vi "SHI_Cryopump_interface_GUI.vi"(8 "error in (no error)":errorcluster, 9 "URL prefex":string, 10 "Http session":T1, 11 "go":bool=TRUE) -> ()   [LabVIEW 2017]
uses:
  Type_Defs/Cryo_Pump_MCC_Status.ctl
  Type_Defs/Cryo_Pump_MCC_CryoPump.ctl
  Type_Defs/Cryo_Pump_MCC_RoughingInterlock.ctl
  Type_Defs/Cryo_Pump_MCC_Status_Status.ctl
  Type_Defs/Cryo_Pump_MCC_Start_Regen.ctl
  Type_Defs/Cryo_Pump_MCC_First_Stage_Temp_CTL.ctl
  Type_Defs/Cryo_Pump_MCC_Params_Power_Failure_Recovery.ctl
  Type_Defs/Cryo_Pump_MCC_Regen_Params.ctl
  Type_Defs/Cryo_Pump_Compressor_Status.ctl
  Type_Defs/Cryo_Pump_Compressor_Status_Status.ctl
  <vilib>/httpClient/ClientHandle.ctl
  Type_Defs/Cryo_Pump_Plots.ctl
  Type_Defs/Cryo_Pump_MCC_Params.ctl
  msg7171_linux.llb/send single message.vi
  msg7171_linux.llb/send multiple messages.vi
  <vilib>/httpClient/POSTBuffer.vi
  <vilib>/httpClient/LabVIEWHTTPClient.lvlib
panel:
  in  "Cold Head Start":bool
  in  "Compressor On":bool
  in  "Roughing_Ilock_Permission":bool
  in  "TC_Pressure_Guage":bool
  in  "Roughing Valve":bool
  in  "Purge Valve":bool
  in  "Send Regen Start":bool
  out "Compressor":T2
  in  "2nd Stage Temp CTL":u32 max=320 step=1
  out "Regen Time":u32
  out "Regen Step Timer":u32
  in  "Regen Start Delay":u32 max=59994 step=1
  in  "Regen Parameters":T4 {"z" max=1 step=1; "G" max=9999 step=1; "C" min=1 max=3 step=1; "A" max=1 step=1; "6" max=80 step=1; "5" max=200 step=1; "4" min=1 max=100 step=1; "3" min=25 max=200 step=1; "2" max=200 step=1; "1" max=9990 step=1; "0" max=59994 step=1}
  out "Regen Cycles":u32
  out "Power Failure Recovery Status":string
  in  "Power Failure Recovery":T5 items=["Disabled", "Enabled", "Enabled only when Stage 2 < Restart Temp."]
  out "MCC Version":string
  out "Last Rate Of Rise Value":u32
  in  "1st Stage Temp Ctl":T6 {"method" items=["ExtHeat", "1st s ctl", "2nd sctl", "Dual"]; "temp" max=320 step=1}
  out "Failed Repurge Cycles":u32
  out "Failed Rate Of Rise Cycles":u32
  out "Elapsed Time":u32
  in  "Start Regen Parameter":T7=enum."Start full regeneration cycle"
  out "MCC Status":T8
  out "Get Params json":string
  out "Get Status json":string
  in  "exit":bool
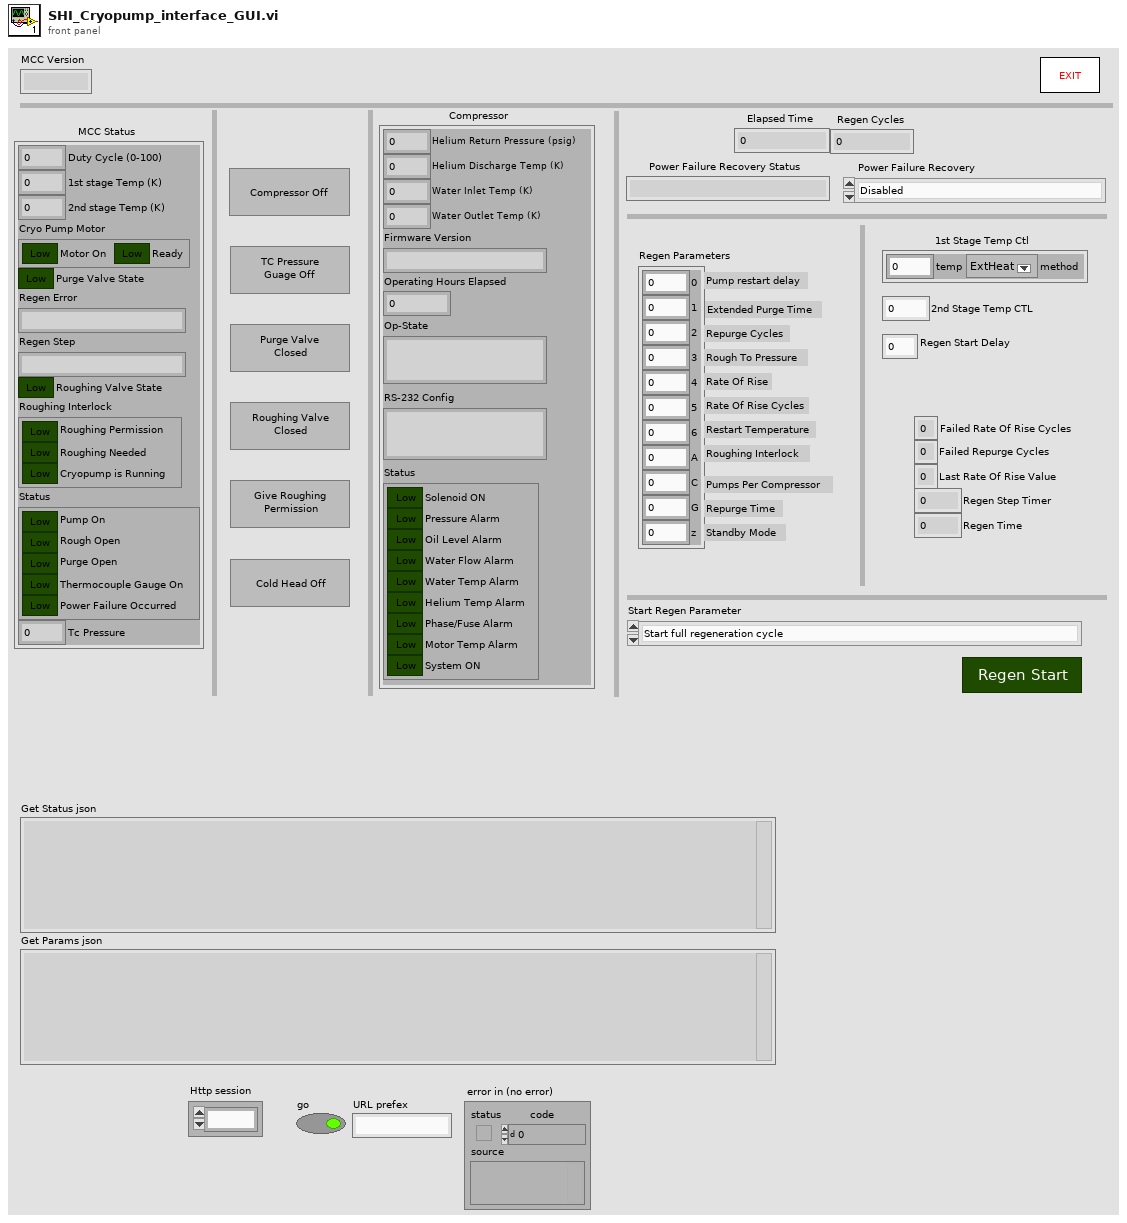
[diagram p1: front panel]
types:
  T1 = typedef "LabVIEWHTTPClient.lvlib/ClientHandle.ctl" = refnum<k1>
  T2 = typedef "Cryo_Pump_Compressor_Status.ctl" = cluster{"Helium Return Pressure (psig)":u32, "Helium Discharge Temp (K)":u32, "Water Inlet Temp (K)":u32, "Water Outlet Temp (K)":u32, "Firmware Version":string, "Operating Hours Elapsed":dbl, "Op-State":string, "RS-232 Config":string, "Status":T3}
  T3 = typedef "Cryo_Pump_Compressor_Status_Status.ctl" = cluster{"Solenoid ON":bool, "Pressure Alarm":bool, "Oil Level Alarm":bool, "Water Flow Alarm":bool, "Water Temp Alarm":bool, "Helium Temp Alarm":bool, "Phase/Fuse Alarm":bool, "Motor Temp Alarm":bool, "System ON":bool}
  T4 = typedef "Cryo_Pump_MCC_Regen_Params.ctl" = cluster{"0":u32, "1":u32, "2":u32, "3":u32, "4":u32, "5":u32, "6":u32, "A":u32, "C":u32, "G":u32, "z":u32}
  T5 = typedef "Cryo_Pump_MCC_Params_Power_Failure_Recovery.ctl" = u16
  T6 = typedef "Cryo_Pump_MCC_First_Stage_Temp_CTL.ctl" = cluster{"temp":u32, "method":u32}
  T7 = typedef "Cryo_Pump_MCC_Start_Regen.ctl" = enum16{"Abort current regeneration cycle", "Start full regeneration cycle", "Start fast regeneration cycle", "Activate stand-by pump module for normal pumping operation", "Warm up cryopump and stop"}
  T8 = typedef "Cryo_Pump_MCC_Status.ctl" = cluster{"Duty Cycle (0-100)":dbl, "1st stage Temp (K)":dbl, "2nd stage Temp (K)":dbl, "Cryo Pump Motor":T9, "Purge Valve State":bool, "Regen Error":string, "Regen Step":string, "Roughing Valve State":bool, "Roughing Interlock":T10, "Status":T11, "Tc Pressure":dbl}
  T9 = typedef "Cryo_Pump_MCC_CryoPump.ctl" = cluster{"Motor On":bool, "Ready":bool}
  T10 = typedef "Cryo_Pump_MCC_RoughingInterlock.ctl" = cluster{"Roughing Permission":bool, "Roughing Needed":bool, "Cryopump is Running":bool}
  T11 = typedef "Cryo_Pump_MCC_Status_Status.ctl" = cluster{"Pump On":bool, "Rough Open":bool, "Purge Open":bool, "Thermocouple Gauge On":bool, "Power Failure Occurred":bool}
  T12 = typedef "Cryo_Pump_Plots.ctl" = cluster{"Duty Cycle (0-100)":dbl, "1st stage Temp (K)":dbl, "2nd stage Temp (K)":dbl, "Helium Return Pressure (psig)":u32, "Helium Discharge Temp (C)":u32, "Water Inlet Temp (C)":u32, "Water Outlet Temp (C)":u32}
  T13 = cluster{"go":bool, "Http session":T1, "URL prefex":string, "Next get param":u32}
  T14 = typedef "Cryo_Pump_MCC_Params.ctl" = cluster{"MCC Version":string, "First Stage Temp CTL":T6, "Second Stage Temp CTL":u32, "Tc Pressure State":bool, "Elapsed Time":u32, "Power Failure Recovery":T5, "Power Failure Recovery Status":string, "Regen Time":u32, "Regen Parameters":T4, "Regen Start Delay":u32, "Regen Step Timer":u32, "Failed Rate Of Rise Cycles":u32, "Failed Repurge Cycles":u32, "Last Rate Of Rise Value":u32, "Regen Cycles":u32}
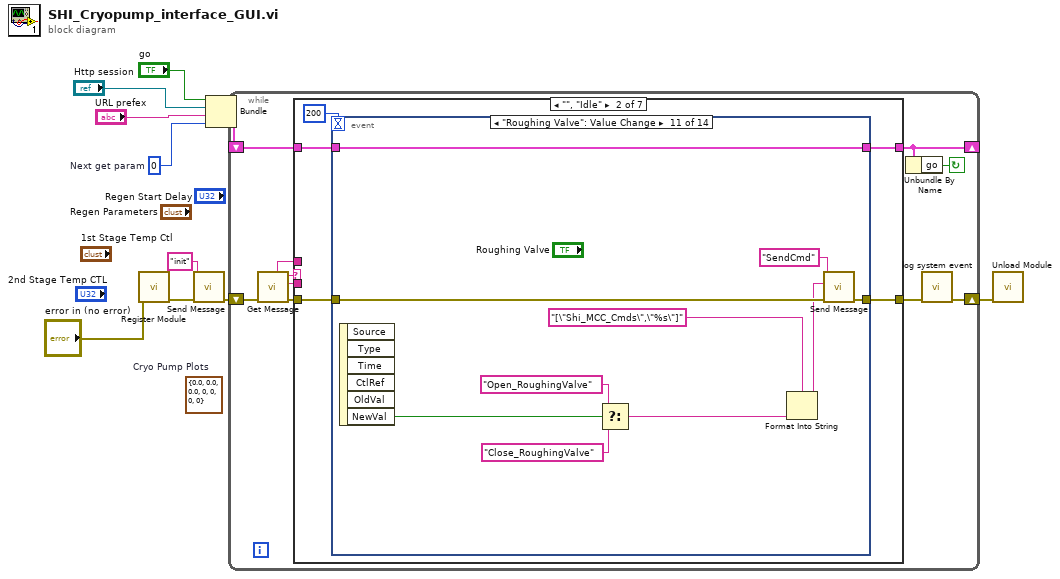
[diagram p0: block diagram]
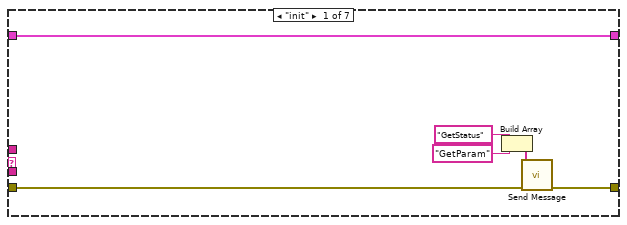
[diagram p2: hidden frame]
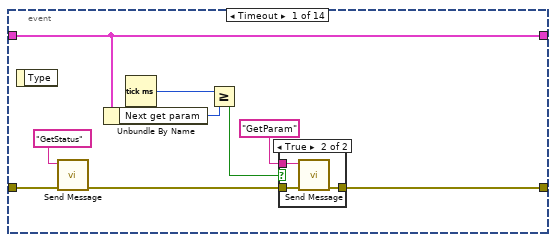
[diagram p3: hidden frame]
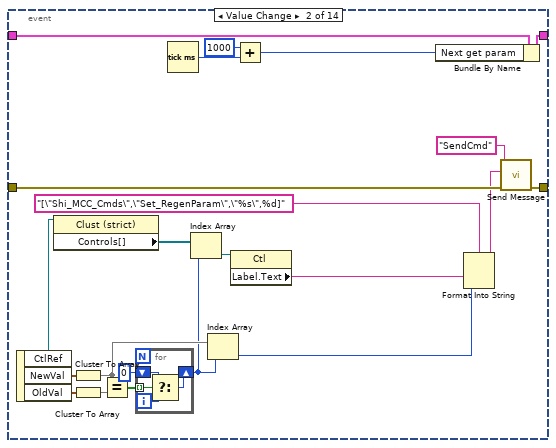
[diagram p5: hidden frame]
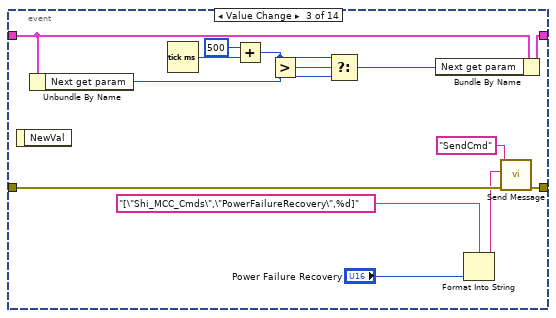
[diagram p6: hidden frame]
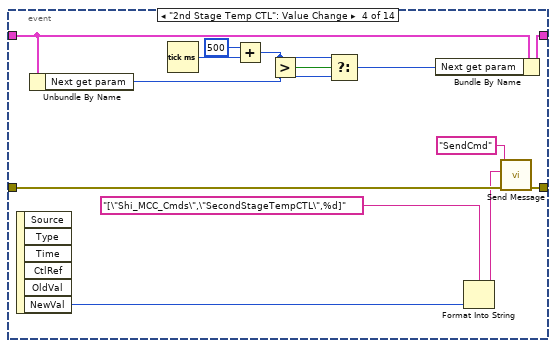
[diagram p7: hidden frame]
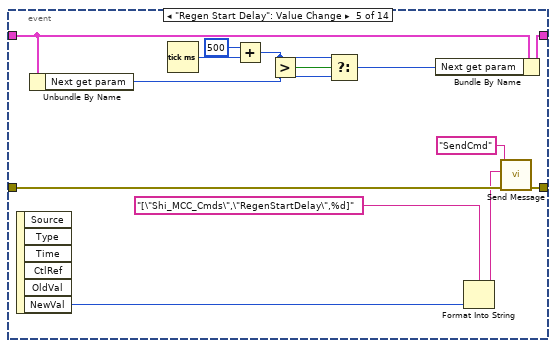
[diagram p8: hidden frame]
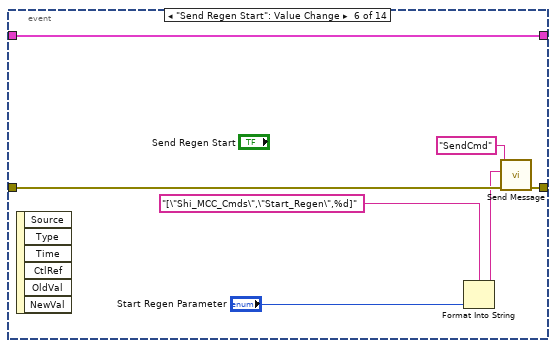
[diagram p9: hidden frame]
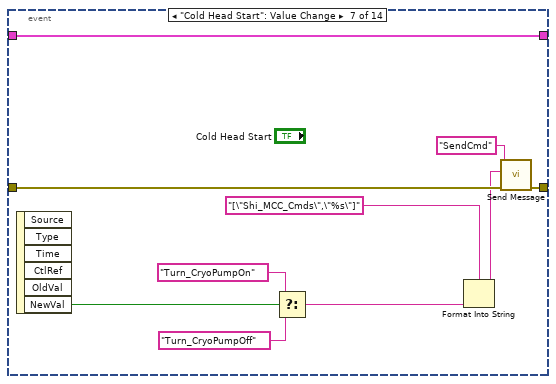
[diagram p10: hidden frame]
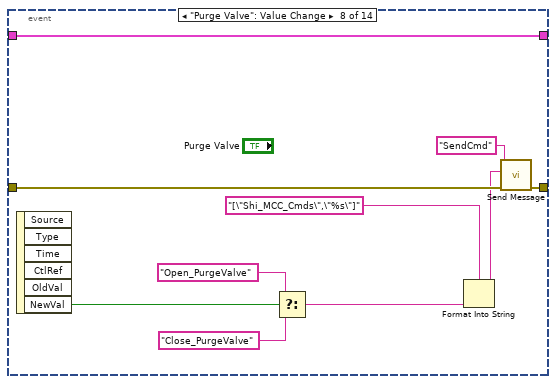
[diagram p11: hidden frame]
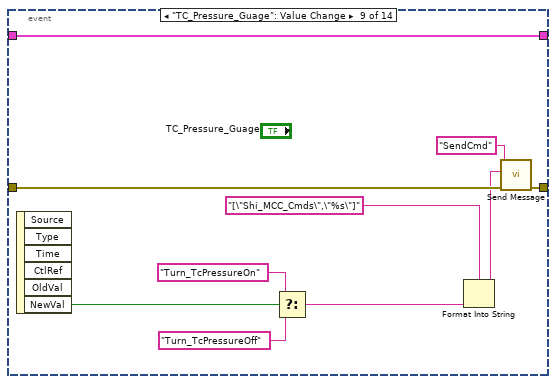
[diagram p12: hidden frame]
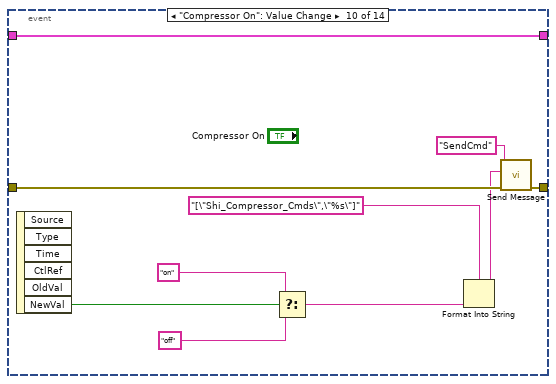
[diagram p13: hidden frame]
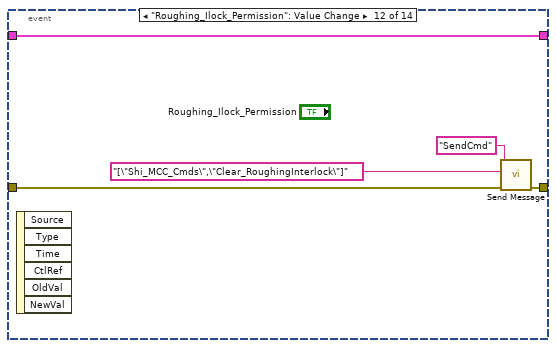
[diagram p14: hidden frame]
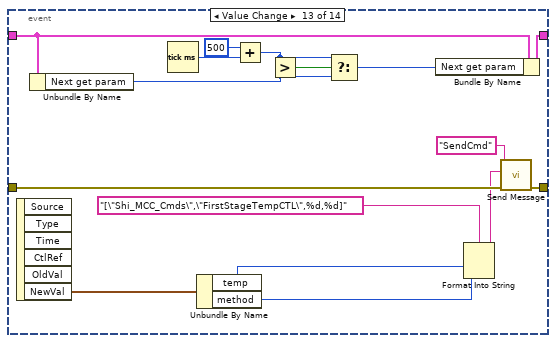
[diagram p15: hidden frame]
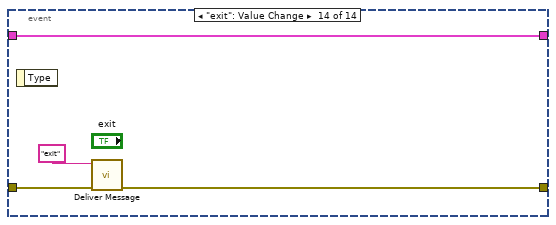
[diagram p16: hidden frame]
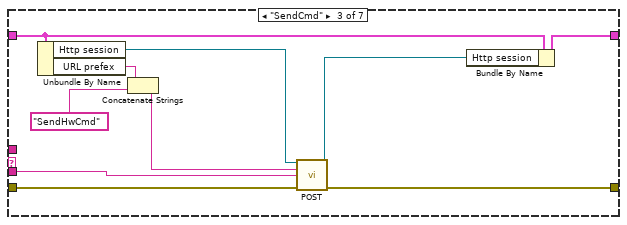
[diagram p17: hidden frame]
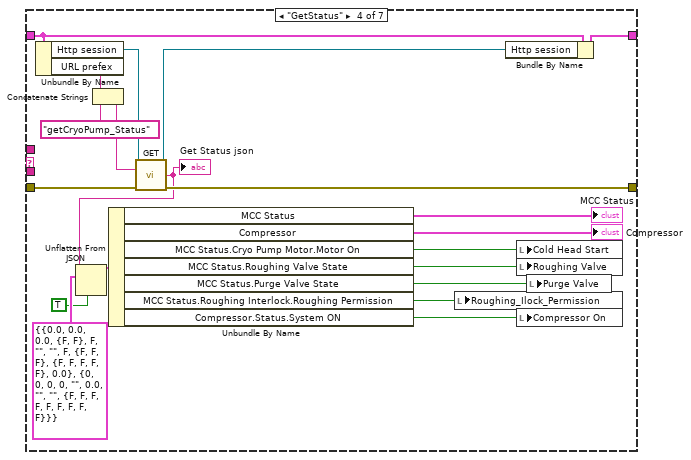
[diagram p18: hidden frame]
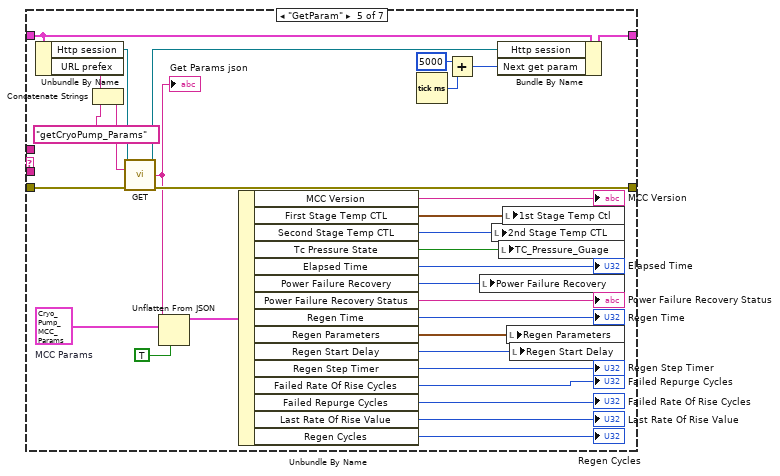
[diagram p19: hidden frame]
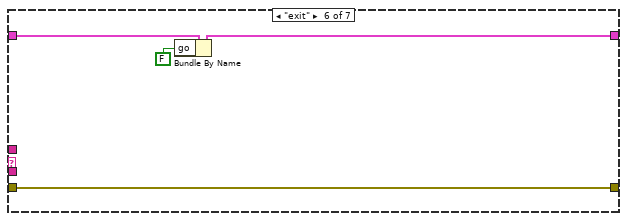
[diagram p20: hidden frame]
diagram:
  (unwired) T12 {"Duty Cycle (0-100)"=0.0, "1st stage Temp (K)"=0.0, "2nd stage Temp (K)"=0.0, "Helium Return Pressure (psig)"=0, "Helium Discharge Temp (C)"=0, "Water Inlet Temp (C)"=0, "Water Outlet Temp (C)"=0}  # Cryo Pump Plots
  w2 = u32 0  # Next get param
  n1 = call "Register Module.vi"("error in (no error)"="error in (no error)") -> ("error out"=w4:errorcluster)  [unwired: 9 in, 1 out]
  n2 = call-poly "Send Message.vi"("error in (no error)"=w4, "event"="init") -> ("error out"=w3:errorcluster)  [unwired: 9 in]
  n3 = Bundle("go"="go", "Http session"="Http session", "URL prefex"="URL prefex", "Next get param"=w2) -> (w10:T13)  [unwired: 1 in]
  n4 = while {
    shift-left: w10 -> [w17]
    shift-right: [w14] -> _
    shift-right: [w12] -> w9
    shift-left: w3 -> [w20]
    stop <- w13 continue-if-true
    n5 = call "Get Message.vi"("error in (no error)"=w20) -> ("error out"=w18:errorcluster, "event buffer"=w19:string, "event"=w16:string, "source"=w15:string)  [unwired: 7 in]
    n6 = case shown="\"\", \"Idle\"" w16 {
      selector: w16 -> [_ _ _ _ _ _ w262]
      tunnel: [w22 w28 w199 w217 w248 w259 w264] -> w14
      tunnel: w17 -> [w22 w27 w198 w216 w247 w257 w264]
      tunnel: w19 -> [_ _ w195 _ _ _ _]
      tunnel: w18 -> [w21 w29 w197 w219 w250 w256 w263]
      tunnel: w15 -> [_ _ _ _ _ _ w261]
      tunnel: [w26 w31 w196 w218 w249 w256 w260] -> w11
      frame "init" {
        n7 = Build Array("GetStatus" ("event"), "GetParam" ("event")) -> (w24:string[])
        n8 = call-poly "Send Message.vi"("error in (no error)"=w21, "event"=w24) -> ("error out"=w26:errorcluster)  [unwired: 9 in]
      }
      frame "", "Idle" {
        n9 = event shown="[10] \"Roughing Valve\": Value Change" {
          selector: _ -> [_ _ _ _ _ _ _ _ _ _ _ _ _ _]
          dyn-events: _ -> [_ _ _ _ _ _ _ _ _ _ _ _ _ _]
          timeout: 200 ("milliseconds to wait") -> [_ _ _ _ _ _ _ _ _ _ _ _ _ _]
          tunnel: w29 -> [w40 w62 w84 w98 w112 w119 w129 w139 w149 w159 w169 w174 w190 w194]
          tunnel: [w36 w61 w83 w97 w111 w118 w128 w138 w148 w158 w168 w173 w189 w193] -> w31
          tunnel: [w32 w48 w78 w92 w106 w113 w120 w130 w140 w150 w160 w170 w184 w191] -> w28
          tunnel: w27 -> [w32 w49 w79 w93 w107 w113 w120 w130 w140 w150 w160 w170 w185 w191]
          event Timeout {
            n10 = event-data() -> ()  [unwired: 1 in, 1 out]
            n11 = call-poly "Send Message.vi"("error in (no error)"=w40, "event"="GetStatus") -> ("error out"=w38:errorcluster)  [unwired: 9 in]
            n12 = Unbundle By Name(w32) -> ("Next get param"=w33:u32)
            n13 = Tick Count (ms)() -> (millisecond timer value=w35:u32)
            n14 = Greater Or Equal?(x=w35, y=w33) -> (x >= y?=w34:bool)
            n15 = case shown="True" w34 {
              tunnel: w38 -> [w41 w44]
              tunnel: [w41 w43] -> w36
              tunnel: "GetParam" ("event") -> [_ w42]
              frame False {
              }
              frame True {
                n16 = call-poly "Send Message.vi"("error in (no error)"=w44, "event"=w42) -> ("error out"=w43:errorcluster)  [unwired: 9 in]
              }
            }
          }
          event Value Change {
            n17 = event-data() -> ("CtlRef"=w53:refnum<vi>, "NewVal"=w63:T4, "OldVal"=w66:T4)  [unwired: 1 in]
            n18 = property class="Clust (strict)"(reference=w53) -> ("Controls[]"=w58:refnum<vi>[])  [unwired: 1 in, 2 out]
            n19 = Cluster To Array(cluster=w63) -> (array=w59:u32[])
            n20 = Cluster To Array(cluster=w66) -> (array=w60:u32[])
            n21 = Equal?(x=w59, y=w60) -> (x = y?=w65:bool[])
            n22 = for {
              tunnel: w65 -> [w70] mode=indexing
              shift-right: [w69] -> w57
              shift-left: 0 -> [w68]
              i -> [w67]
              n23 = Select(t=w68, s=w70, f=w67) -> (s? t:f=w69:i32)
            }
            n24 = Tick Count (ms)() -> (millisecond timer value=w47:u32)
            n25 = Index Array(array=w58, index=w57) -> (element=w56:refnum<vi>)
            n26 = Index Array(array=w59, index=w57) -> (element=w51:u32)
            n27 = property class="Ctl"(reference=w56) -> ("Label.Text"=w50:string)  [unwired: 1 in, 2 out]
            n28 = Add(x=u32 1000, y=w47) -> (x+y=w45:u32)
            n29 = Bundle By Name(cluster=w49, "Next get param"=w45) -> (w48:T13)
            n30 = Format Into String(format string="[\"Shi_MCC_Cmds\",\"Set_RegenParam\",\"%s\",%d]" ("string"), w50, w51) -> (resulting string=w52:string)  [unwired: 2 in, 1 out]
            n31 = call-poly "Send Message.vi"("error in (no error)"=w62, "event buffer"=w52, "event"="SendCmd") -> ("error out"=w61:errorcluster)  [unwired: 8 in]
          }
          event Value Change {
            n32 = event-data() -> ()  [unwired: 1 in, 1 out]
            n33 = Unbundle By Name(w79) -> ("Next get param"=w73:u32)
            n34 = Tick Count (ms)() -> (millisecond timer value=w77:u32)
            n35 = Add(x=u32 500, y=w77) -> (x+y=w72:u32)
            n36 = Greater?(x=w72, y=w73) -> (0:w75:bool)
            n37 = Select(t=w72, s=w75, f=w73) -> (s? t:f=w74:u32)
            n38 = Bundle By Name(cluster=w79, "Next get param"=w74) -> (w78:T13)
            n39 = Format Into String(format string="[\"Shi_MCC_Cmds\",\"PowerFailureRecovery\",%d]" ("string"), "Power Failure Recovery") -> (resulting string=w80:string)  [unwired: 2 in, 1 out]
            n40 = call-poly "Send Message.vi"("error in (no error)"=w84, "event buffer"=w80, "event"="SendCmd") -> ("error out"=w83:errorcluster)  [unwired: 8 in]
          }
          event "2nd Stage Temp CTL": Value Change {
            n41 = event-data() -> ("NewVal"=w85:u32)  [unwired: 1 in, 5 out]
            n42 = Unbundle By Name(w93) -> ("Next get param"=w87:u32)
            n43 = Tick Count (ms)() -> (millisecond timer value=w91:u32)
            n44 = Add(x=u32 500, y=w91) -> (x+y=w86:u32)
            n45 = Greater?(x=w86, y=w87) -> (0:w89:bool)
            n46 = Select(t=w86, s=w89, f=w87) -> (s? t:f=w88:u32)
            n47 = Bundle By Name(cluster=w93, "Next get param"=w88) -> (w92:T13)
            n48 = Format Into String(format string="[\"Shi_MCC_Cmds\",\"SecondStageTempCTL\",%d]" ("string"), w85) -> (resulting string=w94:string)  [unwired: 2 in, 1 out]
            n49 = call-poly "Send Message.vi"("error in (no error)"=w98, "event buffer"=w94, "event"="SendCmd") -> ("error out"=w97:errorcluster)  [unwired: 8 in]
          }
          event "Regen Start Delay": Value Change {
            n50 = event-data() -> ("NewVal"=w99:u32)  [unwired: 1 in, 5 out]
            n51 = Unbundle By Name(w107) -> ("Next get param"=w101:u32)
            n52 = Tick Count (ms)() -> (millisecond timer value=w105:u32)
            n53 = Add(x=u32 500, y=w105) -> (x+y=w100:u32)
            n54 = Greater?(x=w100, y=w101) -> (0:w103:bool)
            n55 = Select(t=w100, s=w103, f=w101) -> (s? t:f=w102:u32)
            n56 = Bundle By Name(cluster=w107, "Next get param"=w102) -> (w106:T13)
            n57 = Format Into String(format string="[\"Shi_MCC_Cmds\",\"RegenStartDelay\",%d]" ("string"), w99) -> (resulting string=w108:string)  [unwired: 2 in, 1 out]
            n58 = call-poly "Send Message.vi"("error in (no error)"=w112, "event buffer"=w108, "event"="SendCmd") -> ("error out"=w111:errorcluster)  [unwired: 8 in]
          }
          event "Send Regen Start": Value Change {
            n59 = event-data() -> ()  [unwired: 1 in, 6 out]
            n60 = Format Into String(format string="[\"Shi_MCC_Cmds\",\"Start_Regen\",%d]" ("string"), "Start Regen Parameter") -> (resulting string=w115:string)  [unwired: 2 in, 1 out]
            n61 = call-poly "Send Message.vi"("error in (no error)"=w119, "event buffer"=w115, "event"="SendCmd") -> ("error out"=w118:errorcluster)  [unwired: 8 in]
          }
          event "Cold Head Start": Value Change {
            n62 = event-data() -> ("NewVal"=w124:bool)  [unwired: 1 in, 5 out]
            n63 = Select(t="Turn_CryoPumpOn", s=w124, f="Turn_CryoPumpOff") -> (s? t:f=w123:string)
            n64 = Format Into String(format string="[\"Shi_MCC_Cmds\",\"%s\"]" ("string"), w123) -> (resulting string=w125:string)  [unwired: 2 in, 1 out]
            n65 = call-poly "Send Message.vi"("error in (no error)"=w129, "event buffer"=w125, "event"="SendCmd") -> ("error out"=w128:errorcluster)  [unwired: 8 in]
          }
          event "Purge Valve": Value Change {
            n66 = event-data() -> ("NewVal"=w134:bool)  [unwired: 1 in, 5 out]
            n67 = Select(t="Open_PurgeValve", s=w134, f="Close_PurgeValve") -> (s? t:f=w133:string)
            n68 = Format Into String(format string="[\"Shi_MCC_Cmds\",\"%s\"]" ("string"), w133) -> (resulting string=w135:string)  [unwired: 2 in, 1 out]
            n69 = call-poly "Send Message.vi"("error in (no error)"=w139, "event buffer"=w135, "event"="SendCmd") -> ("error out"=w138:errorcluster)  [unwired: 8 in]
          }
          event "TC_Pressure_Guage": Value Change {
            n70 = event-data() -> ("NewVal"=w144:bool)  [unwired: 1 in, 5 out]
            n71 = Select(t="Turn_TcPressureOn", s=w144, f="Turn_TcPressureOff") -> (s? t:f=w143:string)
            n72 = Format Into String(format string="[\"Shi_MCC_Cmds\",\"%s\"]" ("string"), w143) -> (resulting string=w145:string)  [unwired: 2 in, 1 out]
            n73 = call-poly "Send Message.vi"("error in (no error)"=w149, "event buffer"=w145, "event"="SendCmd") -> ("error out"=w148:errorcluster)  [unwired: 8 in]
          }
          event "Compressor On": Value Change {
            n74 = event-data() -> ("NewVal"=w154:bool)  [unwired: 1 in, 5 out]
            n75 = Select(t="on", s=w154, f="off") -> (s? t:f=w153:string)
            n76 = Format Into String(format string="[\"Shi_Compressor_Cmds\",\"%s\"]" ("string"), w153) -> (resulting string=w155:string)  [unwired: 2 in, 1 out]
            n77 = call-poly "Send Message.vi"("error in (no error)"=w159, "event buffer"=w155, "event"="SendCmd") -> ("error out"=w158:errorcluster)  [unwired: 8 in]
          }
          event "Roughing Valve": Value Change {
            n78 = event-data() -> ("NewVal"=w164:bool)  [unwired: 1 in, 5 out]
            n79 = Select(t="Open_RoughingValve", s=w164, f="Close_RoughingValve") -> (s? t:f=w163:string)
            n80 = Format Into String(format string="[\"Shi_MCC_Cmds\",\"%s\"]" ("string"), w163) -> (resulting string=w165:string)  [unwired: 2 in, 1 out]
            n81 = call-poly "Send Message.vi"("error in (no error)"=w169, "event buffer"=w165, "event"="SendCmd") -> ("error out"=w168:errorcluster)  [unwired: 8 in]
          }
          event "Roughing_Ilock_Permission": Value Change {
            n82 = event-data() -> ()  [unwired: 1 in, 6 out]
            n83 = call-poly "Send Message.vi"("error in (no error)"=w174, "event buffer"="[\"Shi_MCC_Cmds\",\"Clear_RoughingInterlock\"]" ("string"), "event"="SendCmd") -> ("error out"=w173:errorcluster)  [unwired: 8 in]
          }
          event Value Change {
            n84 = event-data() -> ("NewVal"=w175:T6)  [unwired: 1 in, 5 out]
            n85 = Unbundle By Name(w185) -> ("Next get param"=w179:u32)
            n86 = Tick Count (ms)() -> (millisecond timer value=w183:u32)
            n87 = Unbundle By Name(w175) -> ("temp"=w177:u32, "method"=w176:u32)
            n88 = Add(x=u32 500, y=w183) -> (x+y=w178:u32)
            n89 = Greater?(x=w178, y=w179) -> (0:w181:bool)
            n90 = Select(t=w178, s=w181, f=w179) -> (s? t:f=w180:u32)
            n91 = Bundle By Name(cluster=w185, "Next get param"=w180) -> (w184:T13)
            n92 = Format Into String(format string="[\"Shi_MCC_Cmds\",\"FirstStageTempCTL\",%d,%d]" ("string"), w177, w176) -> (resulting string=w186:string)  [unwired: 2 in, 1 out]
            n93 = call-poly "Send Message.vi"("error in (no error)"=w190, "event buffer"=w186, "event"="SendCmd") -> ("error out"=w189:errorcluster)  [unwired: 8 in]
          }
          event "exit": Value Change {
            n94 = event-data() -> ()  [unwired: 1 in, 1 out]
            n95 = call "Deliver Message.vi"("error in (no error)"=w194, "event"="exit") -> ("error out"=w193:errorcluster)  [unwired: 9 in]
          }
        }
      }
      frame "SendCmd" {
        n96 = Unbundle By Name(w198) -> ("Http session"=w203:T1, "URL prefex"=w201:string)
        n97 = Concatenate Strings(w201, "SendHwCmd" ("url")) -> (w202:string)
        n98 = call-poly <vilib>:"POST.vi"("client handle"=w203, "url"=w202, "buffer"=w195, "error in (no error)"=w197) -> ("client handle out"=w204:T1, "error out"=w196:errorcluster)  [unwired: 8 in, 2 out]
        n99 = Bundle By Name(cluster=w198, "Http session"=w204) -> (w199:T13)
      }
      frame "GetStatus" {
        n100 = Unbundle By Name(w216) -> ("Http session"=w223:T1, "URL prefex"=w221:string)
        n101 = Concatenate Strings(w221, "getCryoPump_Status" ("url")) -> (w222:string)
        n102 = call <vilib>:"GET.vi"("client handle"=w223, "url"=w222, "error in (no error)"=w219) -> ("client handle out"=w224:T1, "body"=w206:string, "error out"=w218:errorcluster)  [unwired: 9 in, 1 out]
        "Get Status json" <- w206
        n103 = Unflatten From JSON(JSON string=w206, type and defaults=cluster{"MCC Status":T8, "Compressor":T2} {"MCC Status"={"Duty Cycle (0-100)"=0.0, "1st stage Temp (K)"=0.0, "2nd stage Temp (K)"=0.0, "Cryo Pump Motor"={"Motor On"=FALSE, "Ready"=FALSE}, "Purge Valve State"=FALSE, "Regen Error"="", "Regen Step"="", "Roughing Valve State"=FALSE, "Roughing Interlock"={"Roughing Permission"=FALSE, "Roughing Needed"=FALSE, "Cryopump is Running"=FALSE}, "Status"={"Pump On"=FALSE, "Rough Open"=FALSE, "Purge Open"=FALSE, "Thermocouple Gauge On"=FALSE, "Power Failure Occurred"=FALSE}, "Tc Pressure"=0.0}, "Compressor"={"Helium Return Pressure (psig)"=0, "Helium Discharge Temp (K)"=0, "Water Inlet Temp (K)"=0, "Water Outlet Temp (K)"=0, "Firmware Version"="", "Operating Hours Elapsed"=0.0, "Op-State"="", "RS-232 Config"="", "Status"={"Solenoid ON"=FALSE, "Pressure Alarm"=FALSE, "Oil Level Alarm"=FALSE, "Water Flow Alarm"=FALSE, "Water Temp Alarm"=FALSE, "Helium Temp Alarm"=FALSE, "Phase/Fuse Alarm"=FALSE, "Motor Temp Alarm"=FALSE, "System ON"=FALSE}}}, default null elements? (F)=TRUE) -> (value=w215:cluster{"MCC Status":T8, "Compressor":T2})  [unwired: 4 in, 1 out]
        n104 = Unbundle By Name(w215) -> ("MCC Status"=→"MCC Status":T8, "Compressor"=→"Compressor":T2, "MCC Status.Cryo Pump Motor.Motor On"=w213:bool, "MCC Status.Roughing Valve State"=w212:bool, "MCC Status.Purge Valve State"=w211:bool, "MCC Status.Roughing Interlock.Roughing Permission"=w210:bool, "Compressor.Status.System ON"=w209:bool)
        n105 = local write "Roughing_Ilock_Permission"(w210) -> ()
        n106 = Bundle By Name(cluster=w216, "Http session"=w224) -> (w217:T13)
        n107 = local write "Cold Head Start"(w213) -> ()
        n108 = local write "Roughing Valve"(w212) -> ()
        n109 = local write "Compressor On"(w209) -> ()
        n110 = local write "Purge Valve"(w211) -> ()
      }
      frame "GetParam" {
        w241 = T14 {"MCC Version"="", "First Stage Temp CTL"={"temp"=0, "method"=0}, "Second Stage Temp CTL"=0, "Tc Pressure State"=FALSE, "Elapsed Time"=0, "Power Failure Recovery"=0, "Power Failure Recovery Status"="", "Regen Time"=0, "Regen Parameters"={"0"=0, "1"=0, "2"=0, "3"=0, "4"=0, "5"=0, "6"=0, "A"=0, "C"=0, "G"=0, "z"=0}, "Regen Start Delay"=0, "Regen Step Timer"=0, "Failed Rate Of Rise Cycles"=0, "Failed Repurge Cycles"=0, "Last Rate Of Rise Value"=0, "Regen Cycles"=0}  # MCC Params
        n111 = Unbundle By Name(w247) -> ("Http session"=w254:T1, "URL prefex"=w252:string)
        n112 = Concatenate Strings(w252, "getCryoPump_Params" ("url")) -> (w253:string)
        n113 = call <vilib>:"GET.vi"("client handle"=w254, "url"=w253, "error in (no error)"=w250) -> ("client handle out"=w255:T1, "body"=w242:string, "error out"=w249:errorcluster)  [unwired: 9 in, 1 out]
        "Get Params json" <- w242
        n114 = Unflatten From JSON(JSON string=w242, type and defaults=w241, default null elements? (F)=TRUE) -> (value=w246:T14)  [unwired: 4 in, 1 out]
        n115 = Unbundle By Name(w246) -> ("MCC Version"=→"MCC Version":string, "First Stage Temp CTL"=w239:T6, "Second Stage Temp CTL"=w240:u32, "Tc Pressure State"=w238:bool, "Elapsed Time"=→"Elapsed Time":u32, "Power Failure Recovery"=w235:T5, "Power Failure Recovery Status"=→"Power Failure Recovery Status":string, "Regen Time"=→"Regen Time":u32, "Regen Parameters"=w236:T4, "Regen Start Delay"=w237:u32, "Regen Step Timer"=→"Regen Step Timer":u32, "Failed Rate Of Rise Cycles"=→"Failed Repurge Cycles":u32, "Failed Repurge Cycles"=→"Failed Rate Of Rise Cycles":u32, "Last Rate Of Rise Value"=→"Last Rate Of Rise Value":u32, "Regen Cycles"=→"Regen Cycles":u32)
        n116 = Tick Count (ms)() -> (millisecond timer value=w245:u32)
        n117 = Add(x=u32 5000, y=w245) -> (x+y=w243:u32)
        n118 = local write "Power Failure Recovery"(w235) -> ()
        n119 = local write "2nd Stage Temp CTL"(w240) -> ()
        n120 = Bundle By Name(cluster=w247, "Http session"=w255, "Next get param"=w243) -> (w248:T13)
        n121 = local write "TC_Pressure_Guage"(w238) -> ()
        n122 = local write "1st Stage Temp Ctl"(w239) -> ()
        n123 = local write "Regen Parameters"(w236) -> ()
        n124 = local write "Regen Start Delay"(w237) -> ()
      }
      frame "exit" {
        n125 = Bundle By Name(cluster=w257, "go"=FALSE ("Bundle Element")) -> (w259:T13)
      }
      frame Default {
        n126 = call "Unknown Message Dialog.vi"("source"=w261, "error in (no error)"=w263, "event name"=w262) -> ("error out"=w260:errorcluster)  [unwired: 8 in]
      }
    }
    n127 = Unbundle By Name(w14) -> ("go"=w13:bool)
    n128 = call "log system event.vi"("error in (no error)"=w11) -> ("error out"=w12:errorcluster)  [unwired: 9 in, 1 out]
  }
  n129 = call "Unload Module.vi"("error in (no error)"=w9) -> ()  [unwired: 10 in, 1 out]
